vi "mules_insertelement2Darray.vi"(10 "new element":u8, 11 "2D array in":dbl[][](array[numeric])) -> (3 "2D array out":dbl[][](array[numeric]))   [LabVIEW 2013]
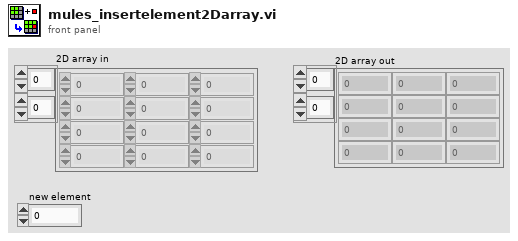
[diagram p1: front panel]
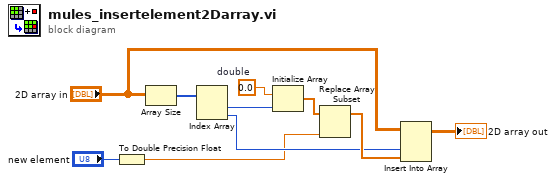
[diagram p0: block diagram]
diagram:
  w9 = 0.0  # double
  n1 = To Double Precision Float(number="new element") -> (double precision float=w1:dbl)
  n2 = Array Size(array="2D array in") -> (size(s)=w10:i32[])
  n3 = Index Array(array=w10) -> (element #1=w7:i32, element #2=w5:i32)  [unwired: 2 in]
  n4 = Initialize Array(w9, w7) -> (w8:dbl[])
  n5 = Replace Array Subset(array=w8, new element=w1) -> (w6:dbl[])  [unwired: 1 in]
  n6 = Insert Into Array(array="2D array in", index (col)=w5, new element=w6) -> (→"2D array out":dbl[][])  [unwired: 1 in]
